vi "文件写入.vi"() -> ()   [LabVIEW 2021]
uses:
  <vilib>/Utility/file.llb/Write Delimited Spreadsheet (string).vi
  <vilib>/Utility/file.llb/Read Delimited Spreadsheet (string).vi
panel:
  in  "工况2文件名":string
  in  "工况1文件名":string
  in  "工况2":string[][](array[string])
  in  "工况1":string[][](array[string])
  in  "探头位置":string[][](array[string])
  out "?":bool
  in  "探头文件名":string
  in  "?":bool
  in  "?":bool
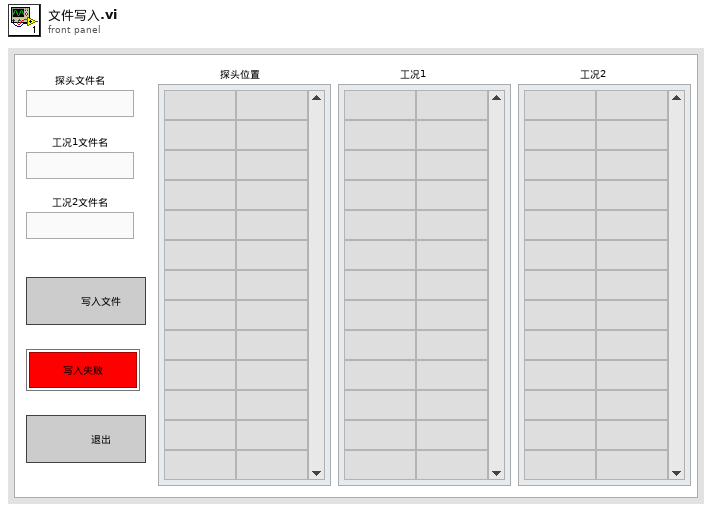
[diagram p1: front panel]
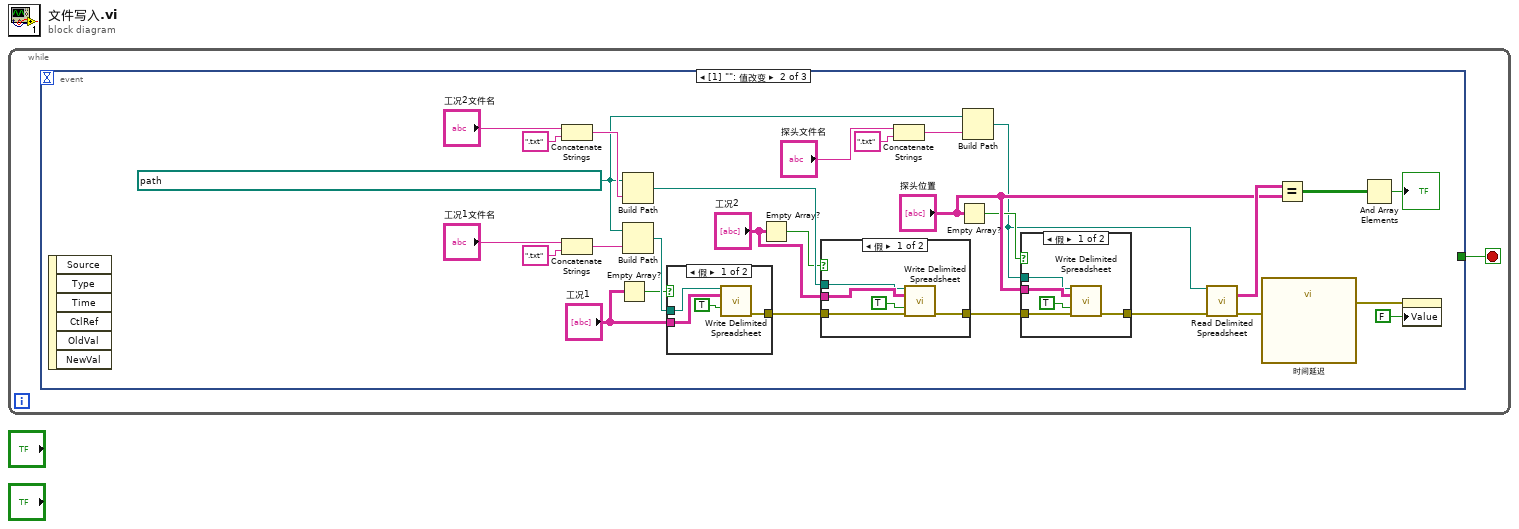
[diagram p0: block diagram]
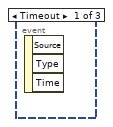
[diagram p2: hidden frame]
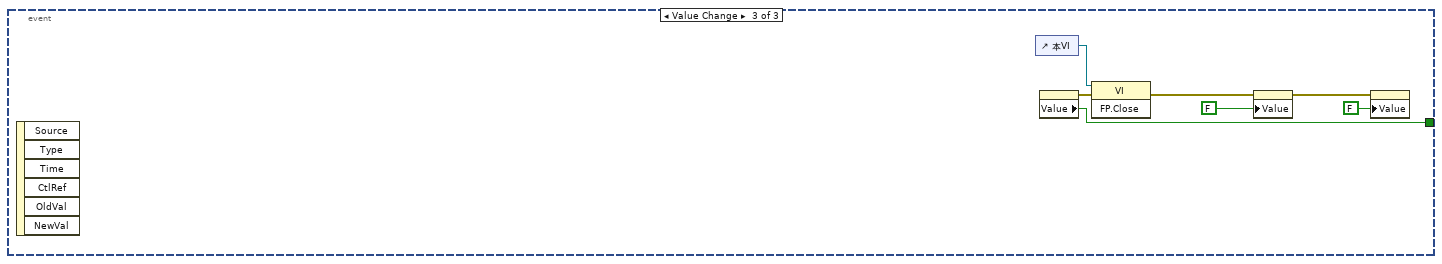
[diagram p6: hidden frame]
diagram:
  n1 = while {
    stop <- w1 stop-if-true
    n2 = event shown="[1] \"\": 值改变" {
      selector: _ -> [_ _ _]
      dyn-events: _ -> [_ _ _]
      timeout: _ -> [_ _ _]
      tunnel: [_ _ w47] -> w1
      event Timeout {
        n3 = event-data() -> ()  [unwired: 1 in, 3 out]
      }
      event Value Change {
        w2 = path "C:/Users/Administrator.CH-202202160008/Desktop/温升测试系统/温升配置文件" ("基路径")
        n4 = event-data() -> ()  [unwired: 1 in, 6 out]
        n5 = Concatenate Strings("工况2文件名", ".txt" ("字符串")) -> (w15:string)
        n6 = Concatenate Strings("工况1文件名", ".txt" ("字符串")) -> (w18:string)
        n7 = Empty Array?(array="工况1") -> (empty?=w10:bool)
        n8 = Build Path(base path=w2, name or relative path=w15) -> (appended path=w13:path)
        n9 = Build Path(base path=w2, name or relative path=w18) -> (appended path=w11:path)
        n10 = case shown="假" w10 {
          tunnel: [w42 _] -> w20
          tunnel: "工况1" -> [w40 _]
          tunnel: w11 -> [w41 _]
          frame False {
            n11 = call-poly <vilib>:"Write Delimited Spreadsheet.vi"("file path (dialog if empty)"=w41, "2D data"=w40, "append to file? (new file:F)"=TRUE) -> ("error out"=w42:errorcluster)  [unwired: 11 in, 1 out]
          }
          frame True {
          }
        }
        n12 = Empty Array?(array="工况2") -> (empty?=w8:bool)
        n13 = case shown="假" w8 {
          tunnel: [w35 _] -> w7
          tunnel: w20 -> [w36 _]
          tunnel: w13 -> [w37 _]
          tunnel: "工况2" -> [w38 _]
          frame False {
            n14 = call-poly <vilib>:"Write Delimited Spreadsheet.vi"("file path (dialog if empty)"=w37, "2D data"=w38, "append to file? (new file:F)"=TRUE, "error in (no error)"=w36) -> ("error out"=w35:errorcluster)  [unwired: 10 in, 1 out]
          }
          frame True {
          }
        }
        n15 = Concatenate Strings("探头文件名", ".txt" ("字符串")) -> (w27:string)
        n16 = Empty Array?(array="探头位置") -> (empty?=w4:bool)
        n17 = Build Path(base path=w2, name or relative path=w27) -> (appended path=w3:path)
        n18 = case shown="假" w4 {
          tunnel: [w30 _] -> w6
          tunnel: w7 -> [w31 _]
          tunnel: w3 -> [w32 _]
          tunnel: "探头位置" -> [w33 _]
          frame False {
            n19 = call-poly <vilib>:"Write Delimited Spreadsheet.vi"("file path (dialog if empty)"=w32, "2D data"=w33, "append to file? (new file:F)"=TRUE, "error in (no error)"=w31) -> ("error out"=w30:errorcluster)  [unwired: 10 in, 1 out]
          }
          frame True {
          }
        }
        n20 = call-poly <vilib>:"Read Delimited Spreadsheet.vi"("file path (dialog if empty)"=w3, "error in (no error)"=w6) -> ("all rows"=w26:string[][], "error out"=w22:errorcluster)  [unwired: 8 in, 4 out]
        n21 = call "时间延迟"("error in (no error)"=w22) -> ("error out"=w21:errorcluster)  [unwired: 10 in]
        n22 = Equal?(x=w26, y="探头位置") -> (x = y?=w25:bool[][])
        n23 = And Array Elements(Boolean array=w25) -> (logical AND=→"?":bool)
        n24 = property class="Bool (严格)"(error in=w21, "Value"=FALSE) -> ()  [unwired: 1 in, 2 out]
      }
      event Value Change {
        n25 = event-data() -> ()  [unwired: 1 in, 6 out]
        n26 = control-ref of="本VI"() -> (w50:refnum<vi>)
        n27 = property class="Bool (严格)"() -> (error out=w46:errorcluster, "Value"=w47:bool)  [unwired: 2 in, 1 out]
        n28 = invoke class="VI" method="FP.Close"(reference=w50, error in=w46) -> (error out=w49:errorcluster)  [unwired: 1 in, 2 out]
        n29 = property class="Bool (严格)"(error in=w49, "Value"=FALSE) -> (error out=w45:errorcluster)  [unwired: 1 in, 1 out]
        n30 = property class="Bool (严格)"(error in=w45, "Value"=FALSE) -> ()  [unwired: 1 in, 2 out]
      }
    }
  }
